vi "test_imu_3d-2.vi"() -> ()   [LabVIEW 2019]
uses:
  Ctrl/cmd_common.ctl
  <vilib>/Instr/_visa.llb/VISA Configure Serial Port (Instr).vi
  <vilib>/picture/3D Picture Control/Object/Create Object (name).vi
  <vilib>/picture/3D Picture Control/NI_3D Picture Control.lvlib
panel:
  out "angle":dbl[](array[numeric])
  out "3D Picture":refnum<vi>(3d-picture)
  in  "Yaw":dbl(knob) scale=0.0..360.0
  in  "Roll":dbl(knob) scale=0.0..360.0
  in  "Pitch":dbl(knob) scale=0.0..360.0
  out "error out":errorcluster caption="에러 출력"
  in  "w":bool
  in  "w-data":string
  out "r buff":u32(graph)
  in  "baud rate":u32=115200 caption="rate"
  in  "Port":refnum<visa-resource-name>="COM24"
  in  "정지":bool
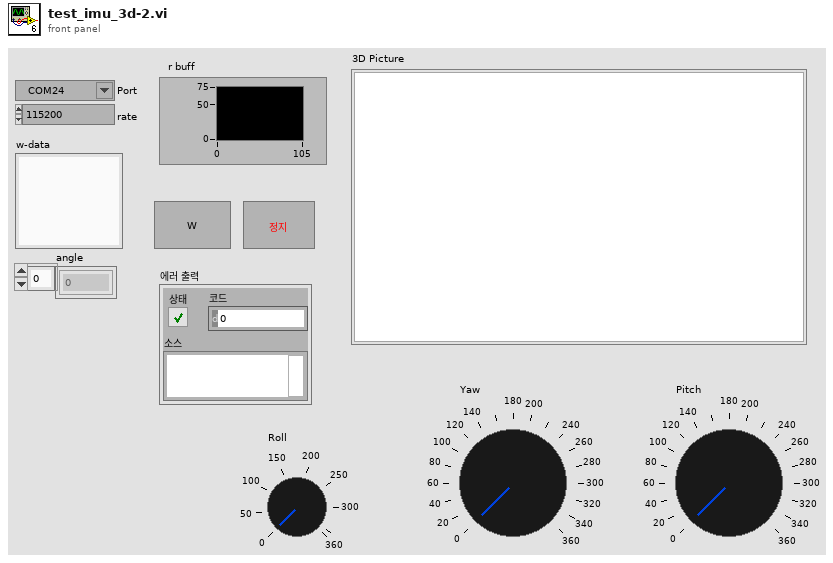
[diagram p1: front panel]
types:
  T1 = typedef "cmd_common.ctl" = enum16{"read", "write"}
  T2 = cluster{"angle":dbl[], "acc":dbl[], "mag":dbl[], "gyr":dbl[]}
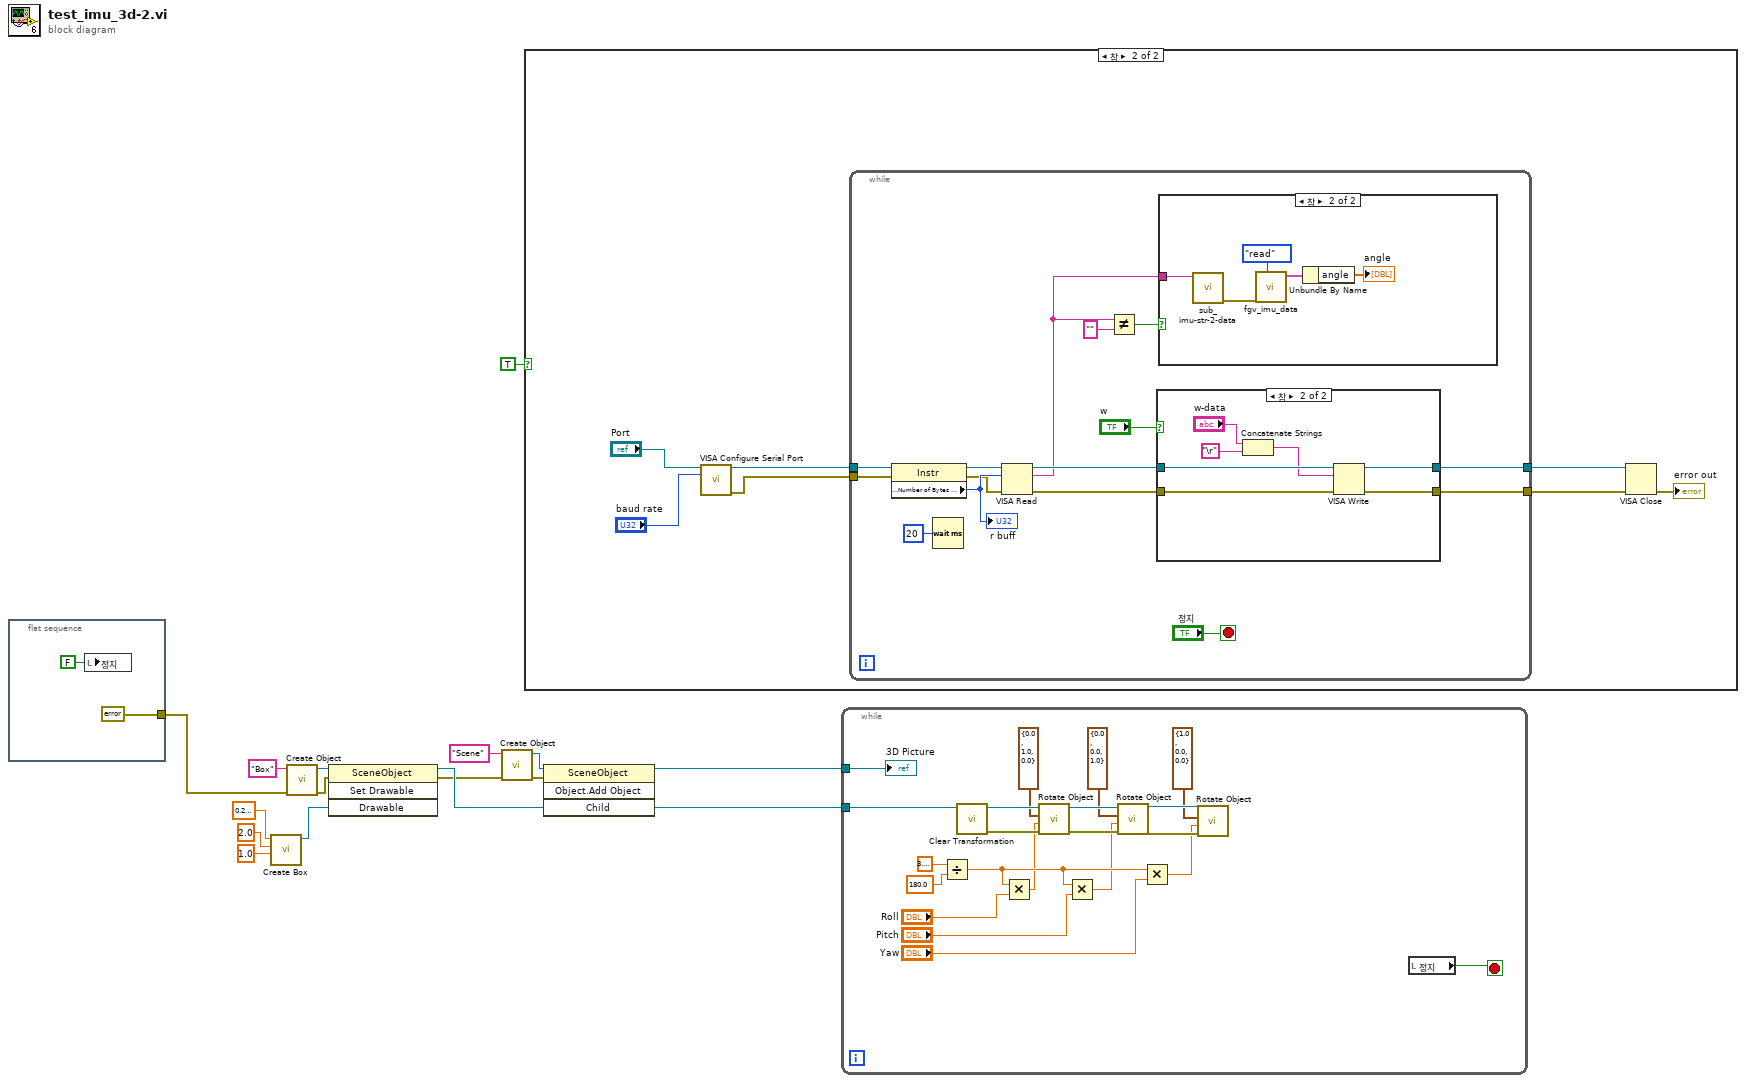
[diagram p0: block diagram]
diagram:
  n1 = flat-sequence {
    tunnel: [errorcluster {"status"=FALSE, "code"=0, "source"=""} ("error in (no error)")] -> w3
    frame #0 {
      n2 = local write "정지"(FALSE ("정지")) -> ()
    }
  }
  n3 = call <vilib>:"Create Box.vi"("Length Z"=sgl 1.0, "Length Y"=sgl 2.0, "Length X"=sgl 0.2) -> ("New Box Refnum"=w12:refnum<vi>)  [unwired: 7 in, 1 out]
  n4 = call-poly <vilib>:"Create Object.vi"("error in (no error)"=w3, "Name"="Box") -> ("error out"=w11:errorcluster, "Scene:New Object"=w10:refnum<vi>)  [unwired: 8 in]
  n5 = invoke class="SceneObject" method="Set Drawable"(reference=w10, error in=w11, "Drawable"=w12) -> (reference out=w16:refnum<vi>, error out=w2:errorcluster)  [unwired: 1 in, 2 out]
  n6 = call-poly <vilib>:"Create Object.vi"("error in (no error)"=w2, "Name"="Scene") -> ("error out"=w15:errorcluster, "Scene:New Object"=w14:refnum<vi>)  [unwired: 8 in]
  n7 = case shown="참" TRUE {
    frame False {
    }
    frame True {
      n8 = call-poly "VISA Configure Serial Port"("VISA resource name"="Port", "baud rate (9600)"="baud rate") -> ("VISA resource name out"=w22:refnum<visa-resource-name>, "error out"=w23:errorcluster)  [unwired: 12 in]
      n9 = while {
        tunnel: w23 -> [w35]
        tunnel: w22 -> [w34]
        tunnel: [w30] -> w20
        tunnel: [w29] -> w19
        stop <- "정지" stop-if-true
        n10 = property class="Instr"(reference=w34, error in=w35) -> (reference out=w39:refnum<visa-resource-name>, error out=w36:errorcluster, "Serial Settings:Number of Bytes at Serial Port"=w37:u32)
        "r buff" <- w37
        n11 = Wait (ms)(milliseconds to wait=u32 20 ("대기 시간 (ms)")) -> ()  [unwired: 1 out]
        n12 = VISA Read(VISA resource name=w39, byte count=w37, error in (no error)=w36) -> (VISA resource name out=w31:refnum<visa-resource-name>, read buffer=w26:string, error out=w32:errorcluster)  [unwired: 1 out]
        n13 = Not Equal?(x=w26, y="") -> (x != y?=w28:bool)
        n14 = case shown="참" "w" {
          tunnel: w31 -> [w47 w54]
          tunnel: [w47 w53] -> w30
          tunnel: w32 -> [w46 w52]
          tunnel: [w46 w51] -> w29
          frame False {
          }
          frame True {
            n15 = Concatenate Strings("w-data", "\r") -> (w48:string)
            n16 = VISA Write(VISA resource name=w54, write buffer=w48, error in (no error)=w52) -> (VISA resource name out=w53:refnum<visa-resource-name>, error out=w51:errorcluster)  [unwired: 1 out]
          }
        }
        n17 = case shown="참" w28 {
          tunnel: w26 -> [_ w45]
          frame False {
          }
          frame True {
            n18 = call "sub_imu-str-2-data.vi"("read buffer"=w45) -> ("error out"=w43:errorcluster)  [unwired: 9 in, 1 out]
            n19 = call "fgv_imu_data.vi"("cmd"=cmd_common."read", "error in"=w43) -> ("IMD data out"=w42:T2)  [unwired: 8 in, 1 out]
            n20 = Unbundle By Name(w42) -> ("angle"=→"angle":dbl[])
          }
        }
      }
      n21 = VISA Close(VISA resource name=w20, error in (no error)=w19) -> (error out=→"error out":errorcluster)
    }
  }
  n22 = invoke class="SceneObject" method="Object.Add Object"(reference=w14, error in=w15, "Child"=w16) -> (reference out=w5:refnum<vi>, "Child"=w4:refnum<vi>)  [unwired: 1 in, 2 out]
  n23 = while {
    tunnel: w5 -> [w62]
    tunnel: w4 -> [w75]
    stop <- w57 stop-if-true
    n24 = Divide(x=3.141592653589793, y=180.0) -> (x/y=w63:dbl)
    n25 = call <vilib>:"Clear Transformation.vi"("Object Refnum In"=w75) -> ("error out"=w71:errorcluster, "Object Refnum Out"=w72:refnum<vi>)  [unwired: 9 in]
    n26 = Multiply(x=w63, y="Roll") -> (x*y=w61:dbl)
    n27 = call <vilib>:"Rotate Object.vi"("error in (no error)"=w71, "Angle"=w61, "Axis"=cluster{"X":sgl, "Y":sgl, "Z":sgl} {"X"=0.0, "Y"=1.0, "Z"=0.0}, "Scene.Object In"=w72) -> ("error out"=w73:errorcluster, "Scene.Object Out"=w74:refnum<vi>)  [unwired: 6 in]
    n28 = Multiply(x=w63, y="Pitch") -> (x*y=w60:dbl)
    n29 = call <vilib>:"Rotate Object.vi"("error in (no error)"=w73, "Angle"=w60, "Axis"=cluster{"X":sgl, "Y":sgl, "Z":sgl} {"X"=0.0, "Y"=0.0, "Z"=1.0}, "Scene.Object In"=w74) -> ("error out"=w66:errorcluster, "Scene.Object Out"=w67:refnum<vi>)  [unwired: 6 in]
    n30 = Multiply(x=w63, y="Yaw") -> (x*y=w56:dbl)
    n31 = call <vilib>:"Rotate Object.vi"("error in (no error)"=w66, "Angle"=w56, "Axis"=cluster{"X":sgl, "Y":sgl, "Z":sgl} {"X"=1.0, "Y"=0.0, "Z"=0.0}, "Scene.Object In"=w67) -> ()  [unwired: 6 in, 2 out]
    n32 = local read "정지"() -> (w57:bool)
    "3D Picture" <- w62
  }
